vi "application.vi"() -> ()   [LabVIEW 2014, in "application.lvclass"]
uses:
  application.lvclass
  application.lvclass/application.ctl
  <vilib>/Utility/config.llb/NI_LVConfig.lvlib
panel:
  in  "Tab Control":enum32{"Main", "Settings"}(tab)
  in  "Settings":bool
  out "CMD":string caption="命令行"
  in  "file path":path=path "D:/Projects/Personal/Multi-LabVIEW-Selector/Multi-LabVIEW Selector.lvproj" caption="打开文件路径"
  in  "LabVIEW List":string(combo)
  in  "OK":bool
  in  "Cancel":bool
  in  "associate file extension":bool
  in  "System Array":string[](array[string]) caption="File Extension"
  in  "Display Time(ms)":i32 min=0 max=10000 step=100
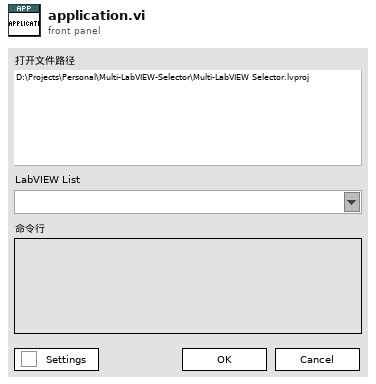
[diagram p1: front panel]
types:
  T1 = enum32{"invalid app kind", "Development System", "Run Time System", "Student Edition", "Embedded LabVIEW", "Evaluation", "Custom"}
  T2 = enum32{"Invalid", "Standard", "Closed", "Hidden", "Minimized", "Maximized"}
  T3 = cluster{"Core":cluster{"Current VI Reference":refnum<vi>, "Close Panel on Exit?":bool}, "RuntimeEngine":bool, "ConfigFilePath":path}
  T4 = cluster{"Current VI Reference":refnum<vi>, "Close Panel on Exit?":bool}
  T5 = typedef "NI_LVConfig.lvlib/Config Data RefNum.ctl" = refnum<k1>
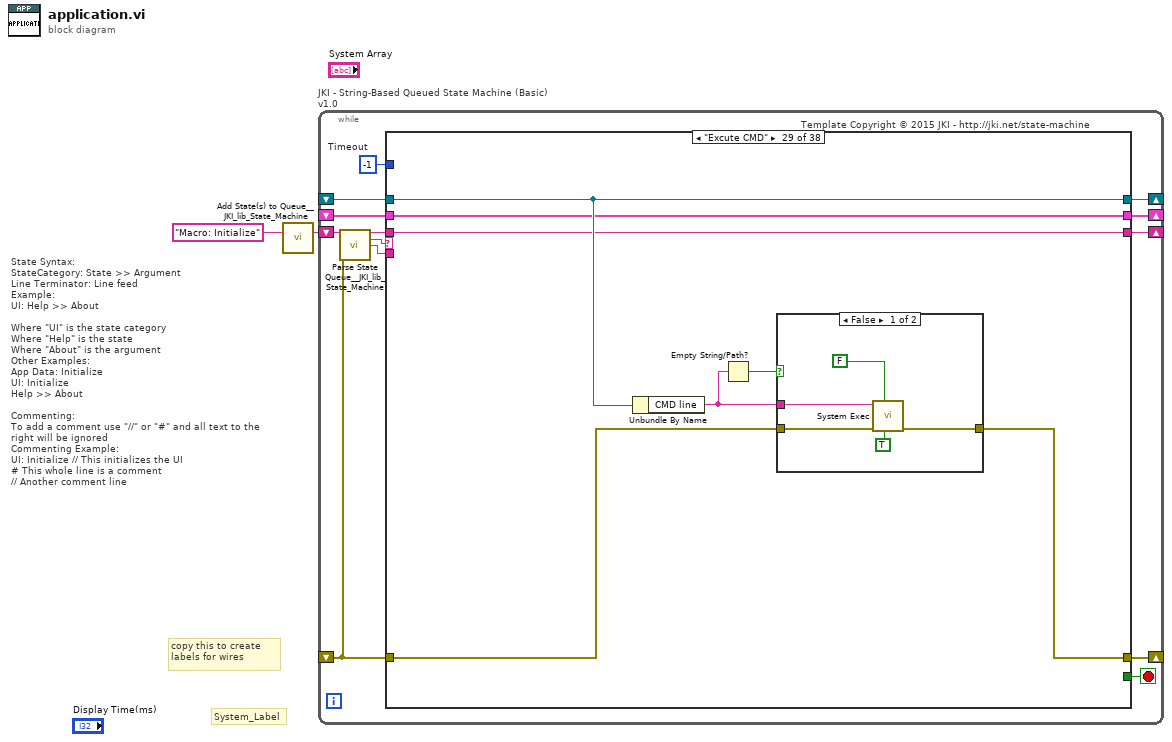
[diagram p0: block diagram]
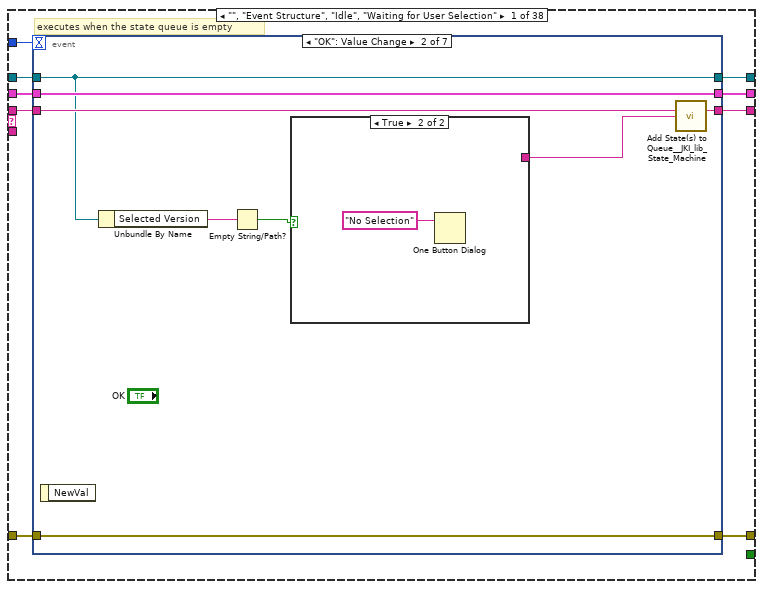
[diagram p2: hidden frame]
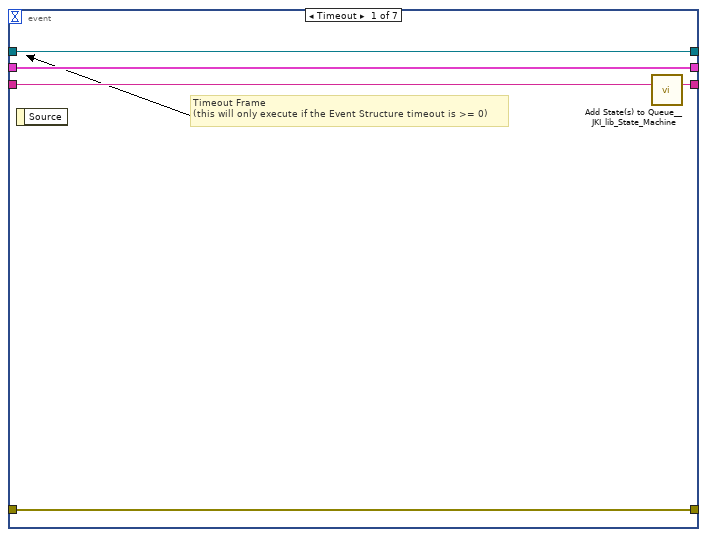
[diagram p3: hidden frame]
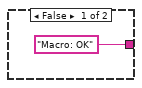
[diagram p4: hidden frame]
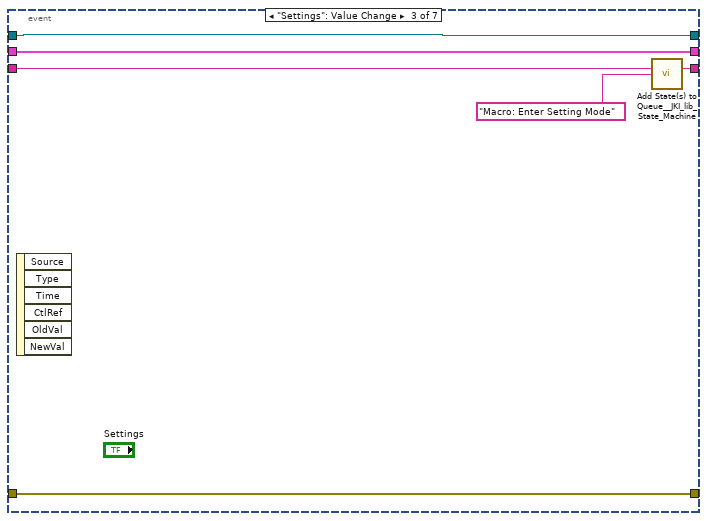
[diagram p5: hidden frame]
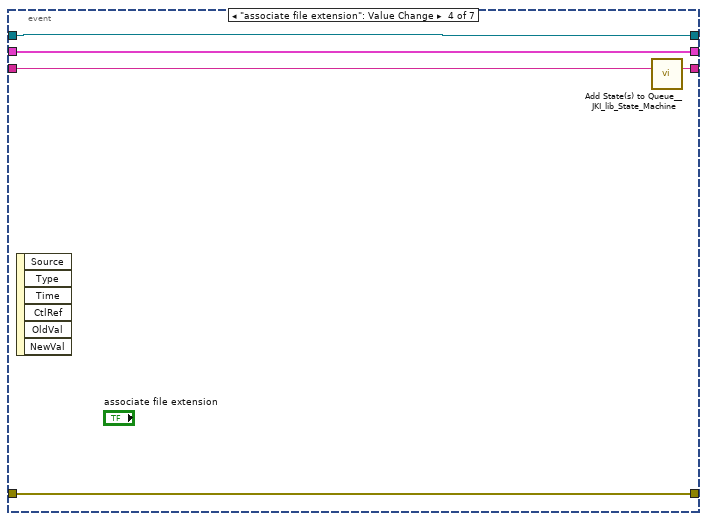
[diagram p6: hidden frame]
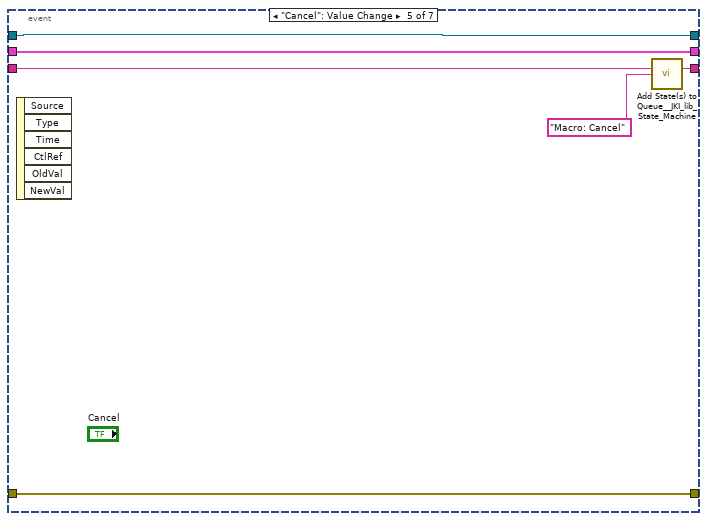
[diagram p7: hidden frame]
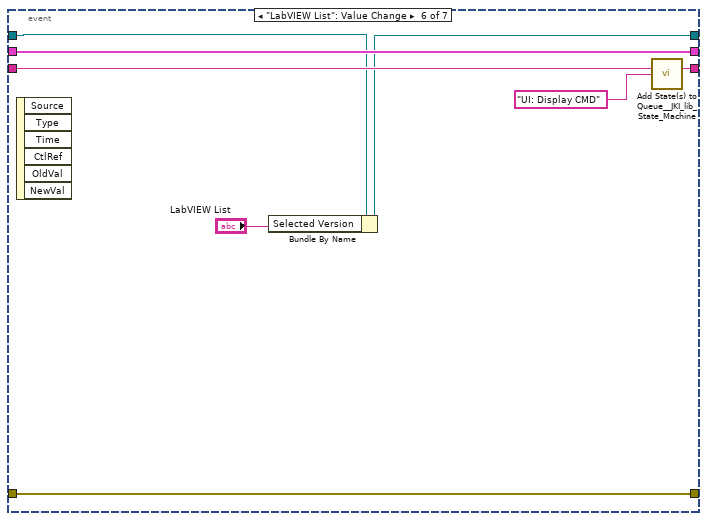
[diagram p8: hidden frame]
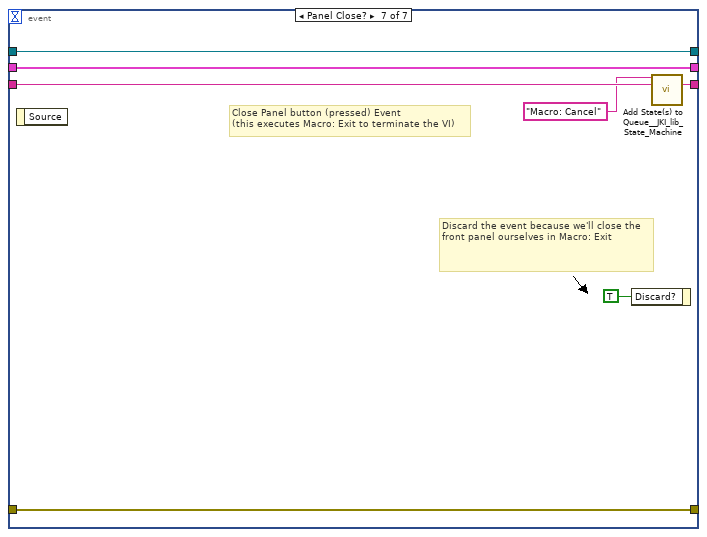
[diagram p9: hidden frame]
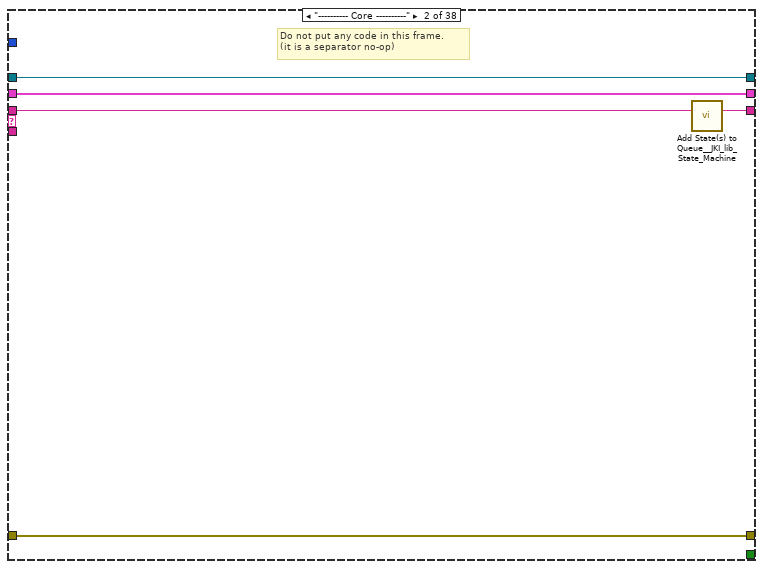
[diagram p10: hidden frame]
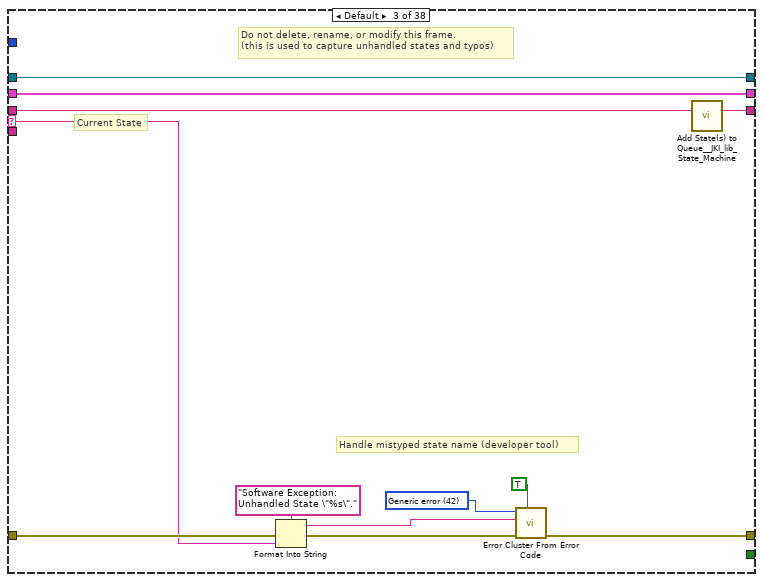
[diagram p11: hidden frame]
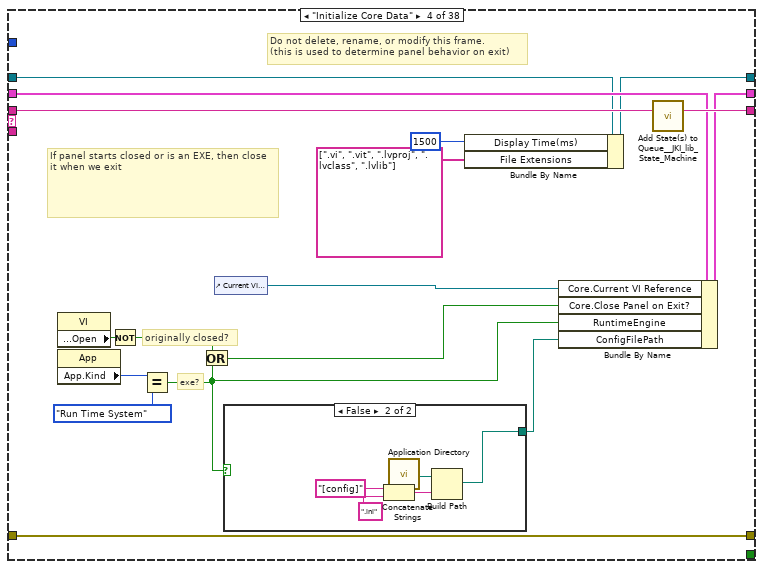
[diagram p12: hidden frame]
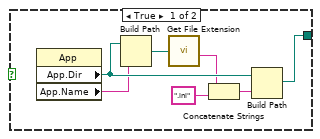
[diagram p13: hidden frame]
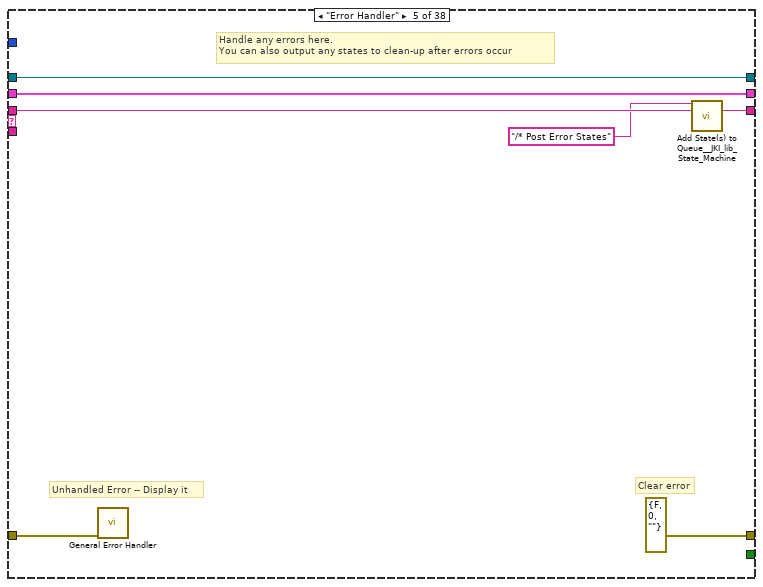
[diagram p14: hidden frame]
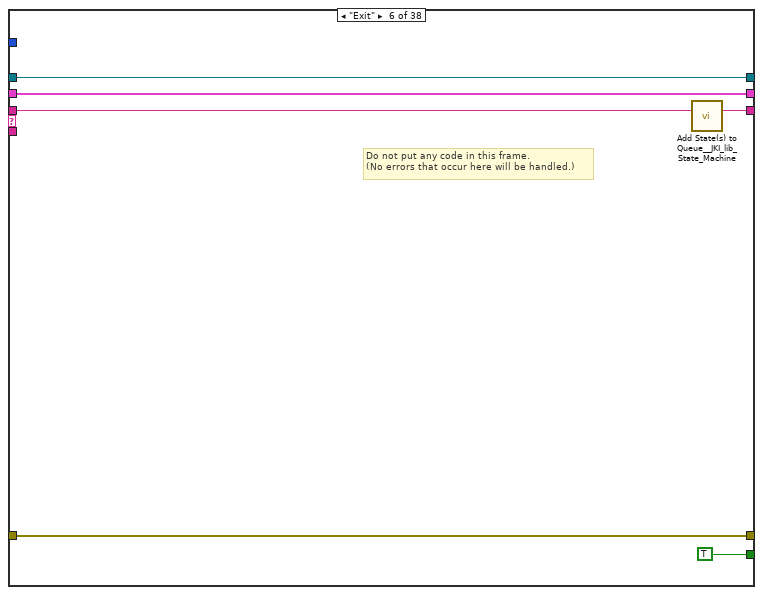
[diagram p15: hidden frame]
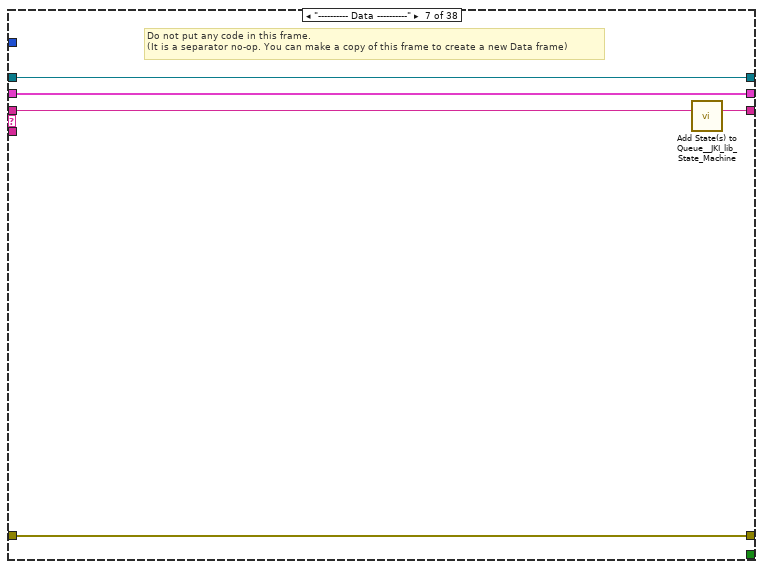
[diagram p16: hidden frame]
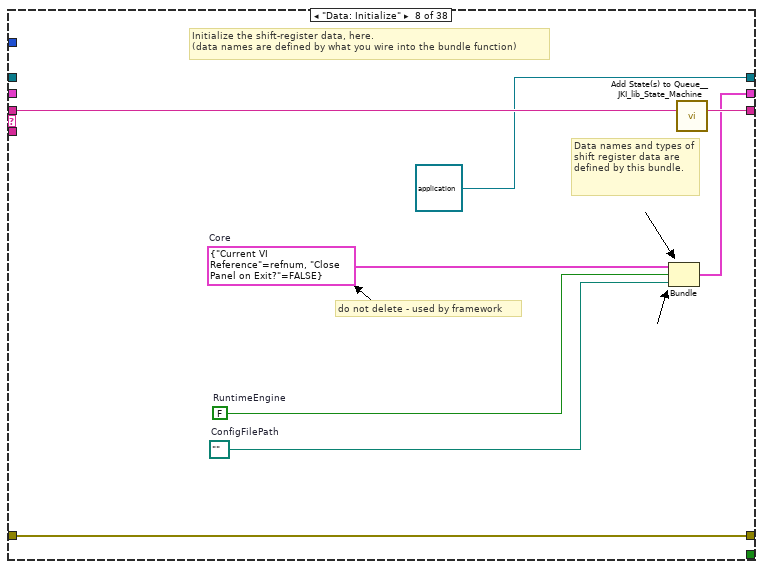
[diagram p17: hidden frame]
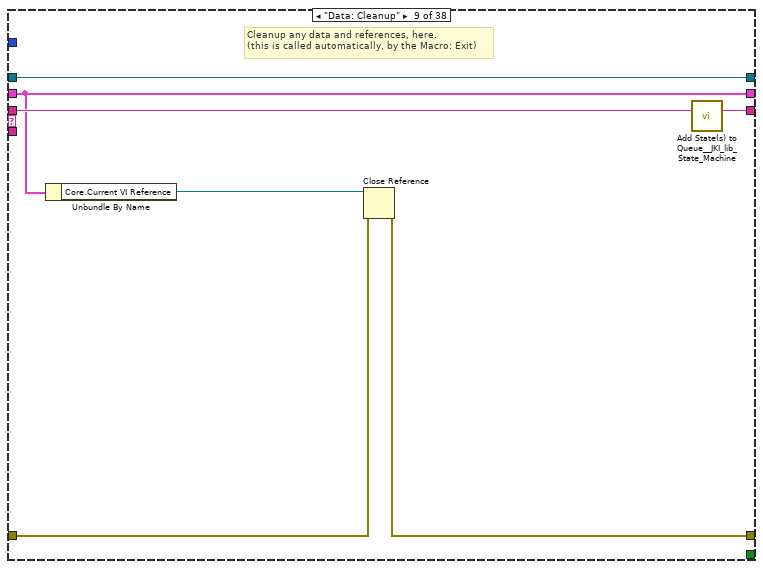
[diagram p18: hidden frame]
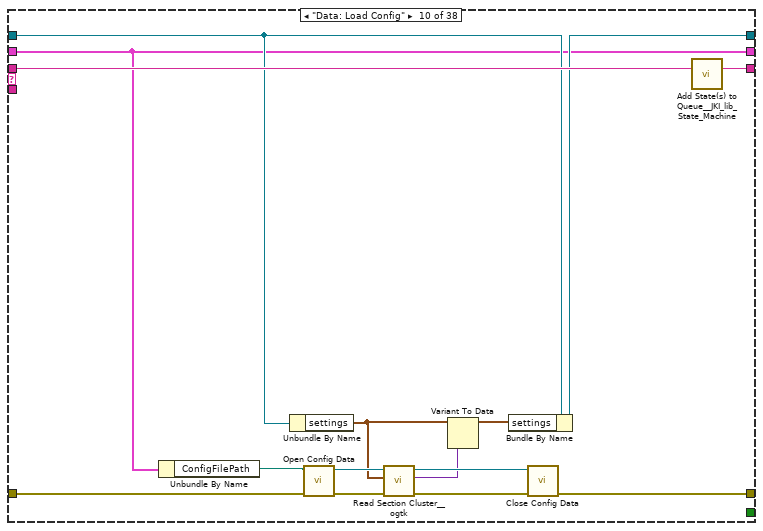
[diagram p19: hidden frame]
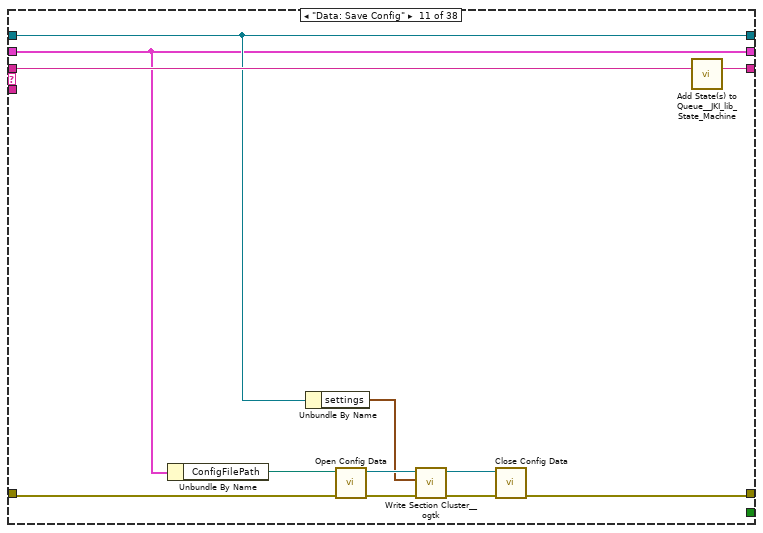
[diagram p20: hidden frame]
diagram:
  # "State Syntax:\nStateCategory: State >> Argument\nLine Terminator: Line feed\nExample:\nUI: Help >> About\n\nWhere \"UI\" is the state category\nWhere \"Help\" is the state\nWhere \"About\" is the argument\nOther Examples:\nApp Data: Initialize\nUI: Initialize\nHelp >> About\n\nCommenting:\nTo add a comment use \"//\" or \"#\" and all text to the right will be ignored\nCommenting Example:\nUI: Initialize // This initializes the UI\n# This whole line is a comment\n// Another comment line"
  # "copy this to create labels for wires"
  # "System_Label"
  n1 = call <vilib>:"Add State(s) to Queue__JKI_lib_State_Machine.vi"("State(s) in (\"\")"="Macro: Initialize") -> ("States Out"=w2:string)  [unwired: 14 in]
  n2 = while "JKI - String-Based Queued State Machine (Basic) v1.0" {
    shift-right: [w8] -> _
    shift-left: _ -> [w7]
    shift-right: [w11] -> _
    shift-left: _ -> [w5]
    shift-right: [w10] -> _
    shift-left: w2 -> [w12]
    shift-right: [w4] -> _
    shift-left: _ -> [w3]
    stop <- w9 stop-if-true
    w6 = -1  # Timeout
    # "Template Copyright © 2015 JKI - http://jki.net/state-machine"
    n3 = call <vilib>:"Parse State Queue__JKI_lib_State_Machine.vi"("State Queue"=w12, "Error In (no error)"=w5) -> ("Remaining States"=w14:string, "Current State"=w15:string, "Arguments"=w13:string)  [unwired: 11 in]
    n4 = case shown="\"Excute CMD\"" w15 {
      selector: w15 -> [_ _ w78 _ _ _ _ _ _ _ _ _ _ _ _ _ _ _ _ _ _ _ _ _ _ _ _ _ _ _ _ _ _ _ _ _ _ _]
      tunnel: w14 -> [w24 w76 w82 w105 w124 w130 w135 w143 w150 w165 w177 w184 w189 w202 w213 w225 w255 w263 w270 w277 w284 w290 w296 w302 w313 w319 w325 w330 w335 w349 w363 w372 w389 w406 w423 w435 w445 w463]
      tunnel: w13 -> [_ _ _ _ _ _ _ _ _ _ _ _ _ _ w208 w219 _ _ _ w272 _ _ _ _ _ _ _ _ _ _ _ _ _ _ _ _ _ _]
      tunnel: w7 -> [w22 w73 w80 w97 w121 w128 w132 _ w145 w152 w166 w182 w186 w200 w211 w221 w253 w260 w267 w274 w281 w287 w293 w299 w310 w316 w322 w327 w336 w345 w360 w368 w391 w408 w425 w437 w447 w465]
      tunnel: [w21 w74 w84 w102 errorcluster {"status"=FALSE, "code"=0, "source"=""} ("error out") w127 w133 w140 w146 w157 w170 w180 w187 w198 w209 w222 w250 w261 w268 w275 w282 w288 w294 w300 w311 w317 w323 w328 w333 w347 w361 w374 w387 w399 w416 w426 w443 w462] -> w11
      tunnel: w5 -> [w20 w74 w83 w102 w120 w127 w133 w140 w147 w158 w169 w181 w187 w196 w210 w223 w251 w261 w268 w275 w282 w288 w294 w300 w311 w317 w323 w328 w334 w348 w361 w375 w387 w400 w417 w427 w444 w462]
      tunnel: [w23 w75 w81 w104 w123 w129 w134 w142 w149 w164 w176 w183 w188 w201 w212 w224 w254 w262 w269 w276 w283 w289 w295 w301 w312 w318 w324 w329 w335 w349 w362 w373 w390 w407 w424 w436 w446 w464] -> w10
      tunnel: [_ _ _ _ _ TRUE _ _ _ _ _ _ _ _ _ _ _ _ _ _ _ _ _ _ _ _ _ _ _ _ _ _ _ _ _ _ _ _] -> w9
      tunnel: [w19 w73 w80 w103 w121 w128 w132 w141 w145 w152 w166 w182 w186 w200 w211 w221 w253 w260 w267 w274 w281 w287 w293 w299 w310 w316 w322 w327 w336 w345 w360 w368 w391 w408 w425 w437 w447 w465] -> w8
      tunnel: w6 -> [w18 _ _ _ _ _ _ _ _ _ _ _ _ _ _ _ _ _ _ _ _ _ _ _ _ _ _ _ _ _ _ _ _ _ _ _ _ _]
      tunnel: [w16 w72 w77 w93 w118 w125 w131 refnum<class "application.lvclass"> refnum ("application.lvclass") w144 w156 w168 w178 w185 w199 w207 w218 w248 w257 w266 w273 w280 w285 w291 w297 w303 w315 w321 w326 w337 w346 w359 w371 w388 w401 w418 w428 w442 w457] -> w4
      tunnel: w3 -> [w17 w72 w77 w94 w118 w125 w131 _ w144 w163 w168 w179 w185 w199 w207 w218 w249 w257 w266 w273 w280 w285 w291 w297 w303 w315 w321 w326 w337 w346 w359 w376 w388 w402 w419 w428 w442 w458]
      frame "", "Event Structure", "Idle", "Waiting for User Selection" {
        # "executes when the state queue is empty"
        n5 = event shown="[1] \"OK\": Value Change" {
          selector: _ -> [_ _ _ _ _ _ _]
          dyn-events: _ -> [_ _ _ _ _ _ _]
          timeout: w18 -> [_ _ _ _ _ _ _]
          tunnel: w24 -> [w29 w37 w45 w50 w56 w64 w71]
          tunnel: [w28 w36 w44 w49 w55 w63 w70] -> w23
          tunnel: w22 -> [w26 w35 w42 w47 w53 w61 w68]
          tunnel: [w27 w34 w43 w48 w54 w62 w69] -> w21
          tunnel: w20 -> [w27 w34 w43 w48 w54 w62 w69]
          tunnel: [w26 w35 w42 w47 w53 w61 w68] -> w19
          tunnel: w17 -> [w25 w33 w41 w46 w52 w60 w65]
          tunnel: [w25 w33 w41 w46 w52 w58 w65] -> w16
          event Timeout {
            # "Timeout Frame\n(this will only execute if the Event Structure timeout is >= 0)"
            n6 = event-data() -> ()  [unwired: 1 in, 1 out]
            n7 = call <vilib>:"Add State(s) to Queue__JKI_lib_State_Machine.vi"("State(s) in (\"\")"=w29) -> ("States Out"=w28:string)  [unwired: 14 in]
          }
          event "OK": Value Change {
            n8 = event-data() -> ()  [unwired: 1 in, 1 out]
            n9 = Unbundle By Name(w33) -> ("Selected Version"=w32:string)
            n10 = Empty String/Path?(string/path=w32) -> (empty?=w31:bool)
            n11 = case shown="True" w31 {
              tunnel: ["Macro: OK" ("State(s) at Back (\"\")") _] -> w30
              frame False {
              }
              frame True {
                n12 = One Button Dialog(message="No Selection") -> ()  [unwired: 1 in, 1 out]
              }
            }
            n13 = call <vilib>:"Add State(s) to Queue__JKI_lib_State_Machine.vi"("State(s) in (\"\")"=w37, "State(s) at Back (\"\")"=w30) -> ("States Out"=w36:string)  [unwired: 13 in]
          }
          event "Settings": Value Change {
            n14 = event-data() -> ()  [unwired: 1 in, 6 out]
            n15 = call <vilib>:"Add State(s) to Queue__JKI_lib_State_Machine.vi"("State(s) in (\"\")"=w45, "State(s) at Back (\"\")"="Macro: Enter Setting Mode" ("State(s) at Back (\"\")")) -> ("States Out"=w44:string)  [unwired: 13 in]
          }
          event "associate file extension": Value Change {
            n16 = event-data() -> ()  [unwired: 1 in, 6 out]
            n17 = call <vilib>:"Add State(s) to Queue__JKI_lib_State_Machine.vi"("State(s) in (\"\")"=w50) -> ("States Out"=w49:string)  [unwired: 14 in]
          }
          event "Cancel": Value Change {
            n18 = event-data() -> ()  [unwired: 1 in, 6 out]
            n19 = call <vilib>:"Add State(s) to Queue__JKI_lib_State_Machine.vi"("State(s) in (\"\")"=w56, "State(s) at Back (\"\")"="Macro: Cancel" ("State(s) at Back (\"\")")) -> ("States Out"=w55:string)  [unwired: 13 in]
          }
          event "LabVIEW List": Value Change {
            n20 = event-data() -> ()  [unwired: 1 in, 6 out]
            n21 = Bundle By Name(cluster=w60, "Selected Version"="LabVIEW List") -> (w58:refnum<class "application.lvclass">)
            n22 = call <vilib>:"Add State(s) to Queue__JKI_lib_State_Machine.vi"("State(s) in (\"\")"=w64, "State(s) at Back (\"\")"="UI: Display CMD" ("State(s) at Back (\"\")")) -> ("States Out"=w63:string)  [unwired: 13 in]
          }
          event Panel Close? {
            # "Discard the event because we'll close the front panel ourselves in Macro: Exit"
            # "Close Panel button (pressed) Event\n(this executes Macro: Exit to terminate the VI)"
            n23 = event-data() -> ()  [unwired: 1 in, 1 out]
            n24 = event-data("Discard?"=TRUE) -> ()  [unwired: 1 in, 1 out]
            n25 = call <vilib>:"Add State(s) to Queue__JKI_lib_State_Machine.vi"("State(s) in Front (\"\")"="Macro: Cancel", "State(s) in (\"\")"=w71) -> ("States Out"=w70:string)  [unwired: 13 in]
          }
        }
      }
      frame "---------- Core ----------" {
        # "Do not put any code in this frame.\n(it is a separator no-op)"
        n26 = call <vilib>:"Add State(s) to Queue__JKI_lib_State_Machine.vi"("State(s) in (\"\")"=w76) -> ("States Out"=w75:string)  [unwired: 14 in]
      }
      frame Default {
        w87 = 42 items=["No error", "Argument error", "Memory is full", "Out of zone", "End of file", "File already open", "Generic file I/O error", "File not found", "File permission error", "Disk is full", "Duplicate path", "Too many files open", "System feature not enabled", "Resource file not found", "Cannot add resource", "Resource not found", "Image not found", "Image memory error", "Pen does not exist", "Config type invalid", "Config token not found", "Config parse error", "Config memory error", "Bad external code format", "Bad external code offset", "External code not present", "Null window", "Destroy window error", "Null menu", "Print aborted", "Bad print record", "Print driver error", "Windows error during printing", "Memory error during printing", "Print dialog error", "Generic print error", "Invalid device refnum", "Device not found", "Device parameter error", "Device unit error", "Cannot open device", "Device call aborted", "Generic error", "Cancelled by user", "Object ID too low", "Object ID too high", "Object not in heap", "Unknown heap", "Unknown object (invalid DefProc)", "Unknown object (DefProc not in table)", "Message out of range", "Invalid (null) method", "Unknown message", "Manager call not supported", "Bad address", "Network operation in progress", "Network operation timed out", "Connection is busy", "Network attribute not supported", "Network error", "Address in use", "System out of memory", "Connection aborted", "Connection refused", "Not connected", "Already connected", "Connection closed", "Initialization error (interapplication manager)", "Bad occurrence", "Wait on unbound occurrence handler", "Occurrence queue overflow", "Datalog type conflict", "Unused", "Unrecognized type (interapplication manager)", "Memory corrupt", "Failed to make temporary DLL", "Old CIN version", "Drag socket not found", "Failed to load drop-object", "Failed to register OLE object", "Failed to release OLE object", "Format specifier type mismatch", "Unknown format specifier", "Too few format specifiers", "Too many format specifiers", "Scan failed", "Newer CIN version", "Error converting to variant", "Runtime menu error", "Password tampered", "Variant attribute not found", "Incompatible variant data type", "Event data is not available", "Event Store is not present", "Occurrence is not found", "Event Queue is not created", "Event info is not available", "Refnum passed is NULL", "Error retrieving Class GUID", "Error retrieving CoClass GUID", "Error retrieving TypeLib GUID.", "Bad built application magic bytes.", "Specific driver is different from the specific driver associated with the Logical Name.", "There is no session opened to the class driver.", "Max Error", "MAX - Error with config objects", "MAX - Error loading configuration", "MAX - Group not supported"]
        # "Current State"
        # "Do not delete, rename, or modify this frame.\n(this is used to capture unhandled states and typos)"
        # "Handle mistyped state name (developer tool)"
        n27 = Format Into String(format string="Software Exception: Unhandled State \"%s\"." ("message"), error in=w83, w78) -> (resulting string=w86:string, error out=w85:errorcluster)  [unwired: 1 in]
        n28 = call <vilib>:"Error Cluster From Error Code.vi"("show call chain? (False)"=TRUE, "error in (no error)"=w85, "error message (\"\")"=w86, "error code (0)"=w87) -> ("error out"=w84:errorcluster)  [unwired: 5 in]
        n29 = call <vilib>:"Add State(s) to Queue__JKI_lib_State_Machine.vi"("State(s) in (\"\")"=w82) -> ("States Out"=w81:string)  [unwired: 14 in]
      }
      frame "Initialize Core Data" {
        # "Do not delete, rename, or modify this frame.\n(this is used to determine panel behavior on exit)"
        # "originally closed?"
        # "exe?"
        # "If panel starts closed or is an EXE, then close it when we exit"
        n30 = property class="VI"() -> ("Front Panel.Open"=w101:bool)  [unwired: 2 in, 2 out]
        n31 = property class="App"() -> ("App.Kind"=w100:T1)  [unwired: 2 in, 2 out]
        n32 = Not(x=w101) -> (.not. x?=w98:bool)
        n33 = Equal?(x=w100, y=T1."Run Time System" ("Application:Kind")) -> (x = y?=w89:bool)
        n34 = Or(x=w98, y=w89) -> (x .or. y?=w96:bool)
        n35 = control-ref of="Current VI Reference"() -> (w95:refnum<vi>)
        n36 = case shown="False" w89 {
          tunnel: [w110 w114] -> w90
          frame True {
            n37 = property class="App"() -> ("App.Dir"=w109:path, "App.Name"=w108:string)  [unwired: 2 in, 2 out]
            n38 = Build Path(base path=w109, name or relative path=w108) -> (appended path=w107:path)
            n39 = call <vilib>:"Get File Extension.vi"("file"=w107) -> ("filename without extension"=w106:string)  [unwired: 7 in, 3 out]
            n40 = Concatenate Strings(w106, ".ini" ("Application:Name")) -> (w111:string)
            n41 = Build Path(base path=w109, name or relative path=w111) -> (appended path=w110:path)
          }
          frame False {
            n42 = Concatenate Strings("[config]" ("string"), ".ini" ("Application:Name")) -> (w115:string)
            n43 = call <vilib>:"Application Directory.vi"() -> ("Application Directory"=w116:path)
            n44 = Build Path(base path=w116, name or relative path=w115) -> (appended path=w114:path)
          }
        }
        n45 = Bundle By Name(cluster=w94, "Display Time(ms)"=1500 ("settings.Display Time(ms)"), "File Extensions"=string[] [".vi", ".vit", ".lvproj", ".lvclass", ".lvlib"]) -> (w93:refnum<class "application.lvclass">)
        n46 = Bundle By Name(cluster=w97, "Core.Current VI Reference"=w95, "Core.Close Panel on Exit?"=w96, "RuntimeEngine"=w89, "ConfigFilePath"=w90) -> (w103:T3)
        n47 = call <vilib>:"Add State(s) to Queue__JKI_lib_State_Machine.vi"("State(s) in (\"\")"=w105) -> ("States Out"=w104:string)  [unwired: 14 in]
      }
      frame "Error Handler" {
        # "Unhandled Error -- Display it"
        # "Handle any errors here.\nYou can also output any states to clean-up after errors occur"
        # "Clear error"
        n48 = call <vilib>:"General Error Handler.vi"("error in (no error)"=w120) -> ()  [unwired: 10 in, 5 out]
        n49 = call <vilib>:"Add State(s) to Queue__JKI_lib_State_Machine.vi"("State(s) in Front (\"\")"="/* Post Error States", "State(s) in (\"\")"=w124) -> ("States Out"=w123:string)  [unwired: 13 in]
      }
      frame "Exit" {
        # "Do not put any code in this frame.\n(No errors that occur here will be handled.)"
        n50 = call <vilib>:"Add State(s) to Queue__JKI_lib_State_Machine.vi"("State(s) in (\"\")"=w130) -> ("States Out"=w129:string)  [unwired: 14 in]
      }
      frame "---------- Data ----------" {
        # "Do not put any code in this frame.\n(It is a separator no-op. You can make a copy of this frame to create a new Data frame)"
        n51 = call <vilib>:"Add State(s) to Queue__JKI_lib_State_Machine.vi"("State(s) in (\"\")"=w135) -> ("States Out"=w134:string)  [unwired: 14 in]
      }
      frame "Data: Initialize" {
        w137 = T4 {"Current VI Reference"=refnum, "Close Panel on Exit?"=FALSE}  # Core
        w139 = FALSE  # RuntimeEngine
        w138 = path ""  # ConfigFilePath
        # "do not delete - used by framework"
        # "Data names and types of shift register data are defined by this bundle."
        # "Initialize the shift-register data, here.\n(data names are defined by what you wire into the bundle function)"
        n52 = Bundle("Core"=w137, "RuntimeEngine"=w139, "ConfigFilePath"=w138) -> (w141:T3)  [unwired: 1 in]
        n53 = call <vilib>:"Add State(s) to Queue__JKI_lib_State_Machine.vi"("State(s) in (\"\")"=w143) -> ("States Out"=w142:string)  [unwired: 14 in]
      }
      frame "Data: Cleanup" {
        # "Cleanup any data and references, here.\n(this is called automatically, by the Macro: Exit)"
        n54 = Unbundle By Name(w145) -> ("Core.Current VI Reference"=w148:refnum<vi>)
        n55 = Close Reference(reference=w148, error in (no error)=w147) -> (error out=w146:errorcluster)
        n56 = call <vilib>:"Add State(s) to Queue__JKI_lib_State_Machine.vi"("State(s) in (\"\")"=w150) -> ("States Out"=w149:string)  [unwired: 14 in]
      }
      frame "Data: Load Config" {
        n57 = Unbundle By Name(w152) -> ("ConfigFilePath"=w151:path)
        n58 = Unbundle By Name(w163) -> ("settings"=w153:cluster{"Display Time(ms)":i32})
        n59 = call <vilib>:"Open Config Data.vi"("error in (no error)"=w158, "configuration file path"=w151) -> ("error out"=w161:errorcluster, "refnum"=w162:T5)  [unwired: 7 in, 1 out]
        n60 = call <userlib>:"Read Section Cluster__ogtk.vi"("error in (no error)"=w161, "Section Formatted Cluster Type"=w153, "refnum"=w162) -> ("error out"=w159:errorcluster, "Section Formatted Cluster"=w154:variant, "dup refnum"=w160:T5)  [unwired: 4 in, 2 out]
        n61 = Variant To Data(type=w153, Variant=w154) -> (data=w155:cluster{"Display Time(ms)":i32})  [unwired: 1 in, 1 out]
        n62 = Bundle By Name(cluster=w163, "settings"=w155) -> (w156:refnum<class "application.lvclass">)
        n63 = call <vilib>:"Close Config Data.vi"("error in (no error)"=w159, "refnum"=w160) -> ("error out"=w157:errorcluster)  [unwired: 8 in, 1 out]
        n64 = call <vilib>:"Add State(s) to Queue__JKI_lib_State_Machine.vi"("State(s) in (\"\")"=w165) -> ("States Out"=w164:string)  [unwired: 14 in]
      }
      frame "Data: Save Config" {
        n65 = Unbundle By Name(w166) -> ("ConfigFilePath"=w167:path)
        n66 = Unbundle By Name(w168) -> ("settings"=w171:cluster{"Display Time(ms)":i32})
        n67 = call <vilib>:"Open Config Data.vi"("error in (no error)"=w169, "configuration file path"=w167) -> ("error out"=w174:errorcluster, "refnum"=w175:T5)  [unwired: 7 in, 1 out]
        n68 = call <userlib>:"Write Section Cluster__ogtk.vi"("error in (no error)"=w174, "Section Formatted Cluster"=w171, "refnum"=w175) -> ("error out"=w172:errorcluster, "dup refnum"=w173:T5)  [unwired: 7 in]
        n69 = call <vilib>:"Close Config Data.vi"("error in (no error)"=w172, "refnum"=w173) -> ("error out"=w170:errorcluster)  [unwired: 8 in, 1 out]
        n70 = call <vilib>:"Add State(s) to Queue__JKI_lib_State_Machine.vi"("State(s) in (\"\")"=w177) -> ("States Out"=w176:string)  [unwired: 14 in]
      }
      frame "Data: Get Installed LabVIEW Version" {
        n71 = call "GetLabVIEWInfos.vi"("error in (no error)"=w181, "application.lvclass"=w179) -> ("error out"=w180:errorcluster, "application.lvclass (dup)"=w178:refnum<class "application.lvclass">)  [unwired: 8 in]
        n72 = call <vilib>:"Add State(s) to Queue__JKI_lib_State_Machine.vi"("State(s) in (\"\")"=w184) -> ("States Out"=w183:string)  [unwired: 14 in]
      }
      frame "---------- UI ----------" {
        # "Do not put any code in this frame.\n(It is a separator no-op. You can make a copy of this frame to create a new UI frame)"
        n73 = call <vilib>:"Add State(s) to Queue__JKI_lib_State_Machine.vi"("State(s) in (\"\")"=w189) -> ("States Out"=w188:string)  [unwired: 14 in]
      }
      frame "UI: Initialize" {
        # "Initialize the User Interface, here.\n(this is called automatically, by the Macro: Init)"
        n74 = disable-structure shown="Default" {
          disable-tunnel: [FALSE ("Tabs Visible?") FALSE ("Tabs Visible?")] -> w195
          disable-tunnel: [w203 w205] -> w194
          disable-tunnel: [w203 w205] -> w193
          frame condition #0 {
            w203 = u32 16777216
          }
          frame condition #1 (active) {
            w205 = u32 16777216
          }
        }
        n75 = property on="Tab Control" class="TabCtl (strict)"(error in=w196, "Tabs Visible?"=w195, "BG Color"=w194, "FG Color"=w193) -> (error out=w191:errorcluster)  [unwired: 1 in, 1 out]
        n76 = property class="VI"(error in=w191, "Front Panel.Title"="Multi-LabVIEW Selector" ("Front Panel Window:Title")) -> (error out=w190:errorcluster)  [unwired: 1 in, 1 out]
        n77 = call <userlib>:"Fit VI window to Content__ogtk.vi"("error in (no error)"=w190, "border spacing (2 px)"=0) -> ("error out"=w198:errorcluster)  [unwired: 4 in, 1 out]
        n78 = call <vilib>:"Add State(s) to Queue__JKI_lib_State_Machine.vi"("State(s) in (\"\")"=w202) -> ("States Out"=w201:string)  [unwired: 14 in]
      }
      frame "UI: Cursor Set" {
        # "Argument"
        # "Set and Unset Cursor Busy.\n(Usage: \"UI: Cursor Set >> Busy|Idle\")"
        n79 = case shown="\"Idle\", Default" w208 {
          tunnel: w210 -> [w215 w217]
          tunnel: [w214 w216] -> w209
          frame "Idle", Default {
            n80 = call <vilib>:"Unset Busy.vi"("error in (no error)"=w215) -> ("error out"=w214:errorcluster)  [unwired: 10 in]
          }
          frame "Busy" {
            n81 = call <vilib>:"Set Busy.vi"("error in (no error)"=w217) -> ("error out"=w216:errorcluster)  [unwired: 9 in, 1 out]
          }
        }
        n82 = call <vilib>:"Add State(s) to Queue__JKI_lib_State_Machine.vi"("State(s) in (\"\")"=w213) -> ("States Out"=w212:string)  [unwired: 14 in]
      }
      frame "UI: Front Panel State" {
        # "Argument"
        # "Set Front Panel Open or Closed\n(Usage: \"UI: Front Panel State >> Open|Close\")"
        n83 = Unbundle By Name(w221) -> ("Core.Current VI Reference"=w220:refnum<vi>)
        n84 = case shown="\"Open\", Default" w219 {
          tunnel: w223 -> [w229 w242]
          tunnel: [w231 w243] -> w222
          tunnel: w220 -> [w230 w240]
          frame "Open", Default {
            n85 = property class="VI"(reference=w230, error in=w229) -> (reference out=w227:refnum<vi>, error out=w228:errorcluster, "Front Panel.Open"=w226:bool)
            n86 = case shown="False" w226 {
              tunnel: [w234 w237] -> w231
              tunnel: w228 -> [w233 w237]
              tunnel: w227 -> [w232 _]
              frame False {
                n87 = invoke class="VI" method="FP.Open"(reference=w232, error in=w233, "Activate"=TRUE, "State"=T2."Standard") -> (error out=w234:errorcluster)  [unwired: 1 in, 4 out]
              }
              frame True {
              }
            }
          }
          frame "Close" {
            n88 = property class="VI"(reference=w240, error in=w242) -> (reference out=w239:refnum<vi>, error out=w241:errorcluster, "Front Panel.Open"=w238:bool)
            n89 = case shown="True" w238 {
              tunnel: [w244 w247] -> w243
              tunnel: w241 -> [w244 w246]
              tunnel: w239 -> [_ w245]
              frame False {
              }
              frame True {
                n90 = invoke class="VI" method="FP.Close"(reference=w245, error in=w246) -> (error out=w247:errorcluster)  [unwired: 1 in, 2 out]
              }
            }
          }
        }
        n91 = call <vilib>:"Add State(s) to Queue__JKI_lib_State_Machine.vi"("State(s) in (\"\")"=w225) -> ("States Out"=w224:string)  [unwired: 14 in]
      }
      frame "UI: Display CMD" {
        n92 = call "GetCMDLine.vi"("error in (no error)"=w251, "application in"=w249) -> ("error out"=w250:errorcluster, "application out"=w248:refnum<class "application.lvclass">)  [unwired: 8 in]
        n93 = Unbundle By Name(w248) -> ("CMD line"=→"CMD":string)
        n94 = call <vilib>:"Add State(s) to Queue__JKI_lib_State_Machine.vi"("State(s) in (\"\")"=w255) -> ("States Out"=w254:string)  [unwired: 14 in]
      }
      frame "UI: Display LabVIEW Information" {
        n95 = Unbundle By Name(w257) -> ("Version List"=w259:string[], "Selected Version"=w258:string)
        n96 = control-ref of="LabVIEW List"() -> (w256:refnum<vi>)
        n97 = property on="Property Node" class="CmbBox"(reference=w256, "Strings[]"=w259, "Value"=w258) -> ()  [unwired: 1 in, 2 out]
        n98 = call <vilib>:"Add State(s) to Queue__JKI_lib_State_Machine.vi"("State(s) in (\"\")"=w263) -> ("States Out"=w262:string)  [unwired: 14 in]
      }
      frame "UI: Display Settings" {
        n99 = Unbundle By Name(w266) -> ("Display Time(ms)"=w265:i32, "File Extensions"=w264:string[])
        n100 = local write "Display Time(ms)"(w265) -> ()
        n101 = local write "System Array"(w264) -> ()
        n102 = call <vilib>:"Add State(s) to Queue__JKI_lib_State_Machine.vi"("State(s) in (\"\")"=w270) -> ("States Out"=w269:string)  [unwired: 14 in]
      }
      frame "UI: Switch Page" {
        n103 = case shown="\"Settings\"" w272 {
          tunnel: [enum32{"Main", "Settings"}."Settings" ("Tab Control") enum32{"Main", "Settings"}."Main" ("Tab Control")] -> w271
          frame "Settings" {
          }
          frame Default {
          }
        }
        n104 = local write "Tab Control"(w271) -> ()
        n105 = call <vilib>:"Add State(s) to Queue__JKI_lib_State_Machine.vi"("State(s) in (\"\")"=w277) -> ("States Out"=w276:string)  [unwired: 14 in]
      }
      frame "---------- Macro ----------" {
        # "Do not put any code in this frame.\n(It is a separator no-op. You can make a copy of this frame to create a new Macro frame)"
        n106 = call <vilib>:"Add State(s) to Queue__JKI_lib_State_Machine.vi"("State(s) in (\"\")"=w284) -> ("States Out"=w283:string)  [unwired: 14 in]
      }
      frame "Macro: Initialize" {
        # "Initialization Macro\n(This is called once, when the VI starts)"
        n107 = call <vilib>:"Add State(s) to Queue__JKI_lib_State_Machine.vi"("State(s) in Front (\"\")"="Data: Initialize\nInitialize Core Data\nData: Load Config\nData: Get Installed LabVIEW Version\nUI: Initialize\nUI: Front Panel State >> Open\nGet Opened File Name\nUI: Display LabVIEW Information\nUI: Display Settings\nUI: Display CMD", "State(s) in (\"\")"=w290) -> ("States Out"=w289:string)  [unwired: 13 in]
      }
      frame "Macro: OK" {
        # "Initialization Macro\n(This is called once, when the VI starts)"
        n108 = call <vilib>:"Add State(s) to Queue__JKI_lib_State_Machine.vi"("State(s) in Front (\"\")"="Update Symbol\nExcute CMD\nMacro: Exit", "State(s) in (\"\")"=w296) -> ("States Out"=w295:string)  [unwired: 13 in]
      }
      frame "Macro: Cancel" {
        # "Initialization Macro\n(This is called once, when the VI starts)"
        n109 = call <vilib>:"Add State(s) to Queue__JKI_lib_State_Machine.vi"("State(s) in Front (\"\")"="Macro: Exit", "State(s) in (\"\")"=w302) -> ("States Out"=w301:string)  [unwired: 13 in]
      }
      frame "Macro: Exit" {
        # "Exit Macro\n(This is called once, when the VI exits)"
        n110 = Unbundle By Name(w310) -> ("Core.Close Panel on Exit?"=w309:bool)
        n111 = Select(t="UI: Front Panel State >> Close", s=w309, f="") -> (s? t:f=w306:string)
        n112 = call <vilib>:"Add State(s) to Queue__JKI_lib_State_Machine.vi"("State(s) in (\"\")"=w306, "State(s) at Back (\"\")"="Data: Save Config\nData: Cleanup\nExit") -> ("States Out"=w304:string)  [unwired: 13 in]
        n113 = call <vilib>:"Add State(s) to Queue__JKI_lib_State_Machine.vi"("State(s) in Front (\"\")"=w304, "State(s) in (\"\")"=w313) -> ("States Out"=w312:string)  [unwired: 13 in]
      }
      frame "Macro: Enter Setting Mode" {
        n114 = call <vilib>:"Add State(s) to Queue__JKI_lib_State_Machine.vi"("State(s) in Front (\"\")"="UI: Switch Page >> Settings" ("State(s) in Front (\"\")"), "State(s) in (\"\")"=w319) -> ("States Out"=w318:string)  [unwired: 13 in]
      }
      frame "Macro: Enter Normal Mode" {
        n115 = call <vilib>:"Add State(s) to Queue__JKI_lib_State_Machine.vi"("State(s) in Front (\"\")"="UI: Switch Page >> Normal\nFind Symbol\nCheck If The Symbol Version Exist" ("State(s) in Front (\"\")"), "State(s) in (\"\")"=w325) -> ("States Out"=w324:string)  [unwired: 13 in]
      }
      frame "---------- State Machine ----------" {
        n116 = call <vilib>:"Add State(s) to Queue__JKI_lib_State_Machine.vi"("State(s) in (\"\")"=w330) -> ("States Out"=w329:string)  [unwired: 14 in]
      }
      frame "Excute CMD" {
        n117 = Unbundle By Name(w337) -> ("CMD line"=w331:string)
        n118 = Empty String/Path?(string/path=w331) -> (empty?=w332:bool)
        n119 = case shown="False" w332 {
          tunnel: w331 -> [w340 _]
          tunnel: w334 -> [w339 w343]
          tunnel: [w338 w343] -> w333
          frame False {
            n120 = call <vilib>:"System Exec.vi"("run minimized? (F)"=TRUE, "wait until completion? (T)"=FALSE, "error in (no error)"=w339, "command line"=w340) -> ("error out"=w338:errorcluster)  [unwired: 4 in, 3 out]
          }
          frame True {
          }
        }
      }
      frame "Associate with File Extension" {
        n121 = Unbundle By Name(w345) -> ("RuntimeEngine"=w344:bool)
        n122 = case shown="True" w344 {
          tunnel: w348 -> [w350 w354]
          tunnel: [w350 w353] -> w347
          tunnel: w346 -> [_ w352]
          frame False {
          }
          frame True {
            n123 = Unbundle By Name(w352) -> ("File Extensions"=w351:string[])
            n124 = for {
              tunnel: w354 -> [w358]
              tunnel: [w357] -> w353
              tunnel: w351 -> [w356] mode=indexing
              n125 = call "Associate a File Extension.vi"("error in (no error)"=w358, "string"=w356, "exe path"=path "") -> ("error out"=w357:errorcluster)  [unwired: 8 in]
            }
          }
        }
      }
      frame "---------- Actions ----------" {
        n126 = call <vilib>:"Add State(s) to Queue__JKI_lib_State_Machine.vi"("State(s) in (\"\")"=w363) -> ("States Out"=w362:string)  [unwired: 14 in]
      }
      frame "Get Opened File Name" {
        n127 = Unbundle By Name(w368) -> ("RuntimeEngine"=w369:bool)
        n128 = case shown="False" w369 {
          tunnel: w375 -> [w377 w385]
          tunnel: [w377 w384] -> w374
          tunnel: ["file path" w383] -> w370
          tunnel: [FALSE w382] -> w367
          frame False {
          }
          frame True {
            n129 = property class="App"(error in=w385) -> (error out=w384:errorcluster, "App.Args"=w381:string[])  [unwired: 1 in, 1 out]
            n130 = Index Array(array=w381) -> (element #2=w380:string)  [unwired: 2 in, 1 out]
            n131 = String To Path(string=w380) -> (path=w383:path)
            n132 = Empty String/Path?(string/path=w383) -> (empty?=w382:bool)
          }
        }
        n133 = Bundle By Name(cluster=w376, "File Path"=w370) -> (w371:refnum<class "application.lvclass">)
        n134 = Select(t="Macro: Enter Setting Mode", s=w367, f="Macro: Enter Normal Mode") -> (s? t:f=w364:string)
        n135 = call <vilib>:"Add State(s) to Queue__JKI_lib_State_Machine.vi"("State(s) in Front (\"\")"=w364, "State(s) in (\"\")"=w372) -> ("States Out"=w373:string)  [unwired: 13 in]
      }
      frame "Find Symbol" {
        n136 = call <vilib>:"Add State(s) to Queue__JKI_lib_State_Machine.vi"("State(s) in Front (\"\")"="Find New Symbol" ("State(s) at Back (\"\")"), "State(s) in (\"\")"=w389) -> ("States Out"=w390:string)  [unwired: 13 in]
      }
      frame "Find New Symbol" {
        n137 = Unbundle By Name(w402) -> ("File Path"=w405:path)
        n138 = Strip Path(path=w405) -> (stripped path=w393:path)  [unwired: 1 out]
        n139 = call "FindSymbol.vi"("error in (no error)"=w400, "pattern"="DEV ENVIRONMENT *" ("prefix"), "path"=w393) -> ("error out"=w399:errorcluster, "Version"=w404:string, "Exits?"=w392:bool, "Symbol path"=w394:path)  [unwired: 4 in, 1 out]
        n140 = Select(t=w394, s=w392, f=w393) -> (s? t:f=w395:path)
        n141 = Bundle By Name(cluster=w402, "Symbol Path"=w395, "Symbol Version"=w404, "Symbol Found?"=w392) -> (w401:refnum<class "application.lvclass">)
        n142 = Select(t="", s=w392, f="Find Old Symbol" ("State(s) at Back (\"\")")) -> (s? t:f=w396:string)
        n143 = call <vilib>:"Add State(s) to Queue__JKI_lib_State_Machine.vi"("State(s) in Front (\"\")"=w396, "State(s) in (\"\")"=w406) -> ("States Out"=w407:string)  [unwired: 13 in]
      }
      frame "Find Old Symbol" {
        # "If old symbol is found, replace with new symbol."
        n144 = Unbundle By Name(w419) -> ("File Path"=w422:path)
        n145 = Strip Path(path=w422) -> (stripped path=w412:path)  [unwired: 1 out]
        n146 = call "FindSymbol.vi"("error in (no error)"=w417, "pattern"="开发环境 *" ("prefix"), "path"=w412) -> ("error out"=w416:errorcluster, "Version"=w421:string, "Exits?"=w409:bool, "Symbol path"=w410:path)  [unwired: 4 in, 1 out]
        n147 = Select(t=w410, s=w409, f=w412) -> (s? t:f=w411:path)
        n148 = Bundle By Name(cluster=w419, "Symbol Path"=w411, "Symbol Version"=w421, "Symbol Found?"=w409) -> (w418:refnum<class "application.lvclass">)
        n149 = Select(t="Replace with New Symbol", s=w409, f="" ("State(s) at Back (\"\")")) -> (s? t:f=w413:string)
        n150 = call <vilib>:"Add State(s) to Queue__JKI_lib_State_Machine.vi"("State(s) in Front (\"\")"=w413, "State(s) in (\"\")"=w423) -> ("States Out"=w424:string)  [unwired: 13 in]
      }
      frame "Replace with New Symbol" {
        n151 = Unbundle By Name(w428) -> ("Symbol Version"=w430:string, "Symbol Path"=w434:path)
        n152 = call "DeleteSymbolsInDir.vi"("error in (no error)"=w427, "pattern"="开发环境 *", "dup path"=w434) -> ("error in (no error) (dup)"=w432:errorcluster, "dup path (dup)"=w431:path)  [unwired: 7 in]
        n153 = call "CreateSymbolInDir.vi"("error in"=w432, "prefix"="DEV ENVIRONMENT", "Name"=w430, "Path"=w431) -> ("error out"=w426:errorcluster)  [unwired: 6 in, 1 out]
        n154 = call <vilib>:"Add State(s) to Queue__JKI_lib_State_Machine.vi"("State(s) in (\"\")"=w435) -> ("States Out"=w436:string)  [unwired: 14 in]
      }
      frame "Update Symbol" {
        n155 = Unbundle By Name(w442) -> ("Symbol Version"=w440:string, "Selected Version"=w439:string, "Symbol Path"=w441:path)
        n156 = Not Equal?(x=w440, y=w439) -> (x != y?=w438:bool)
        n157 = case shown="True" w438 {
          tunnel: w444 -> [w448 w449]
          tunnel: [w448 w456] -> w443
          tunnel: w441 -> [_ w453]
          tunnel: w439 -> [_ w455]
          frame False {
          }
          frame True {
            n158 = call "DeleteSymbolsInDir.vi"("error in (no error)"=w449, "pattern"="DEV ENVIRONMENT*" ("prefix"), "dup path"=w453) -> ("error in (no error) (dup)"=w450:errorcluster, "dup path (dup)"=w452:path)  [unwired: 7 in]
            n159 = call "CreateSymbolInDir.vi"("error in"=w450, "prefix"="DEV ENVIRONMENT", "Name"=w455, "Path"=w452) -> ("error out"=w456:errorcluster)  [unwired: 6 in, 1 out]
          }
        }
        n160 = call <vilib>:"Add State(s) to Queue__JKI_lib_State_Machine.vi"("State(s) in (\"\")"=w445) -> ("States Out"=w446:string)  [unwired: 14 in]
      }
      frame "Check If The Symbol Version Exist" {
        n161 = Unbundle By Name(w458) -> ("Symbol Found?"=w461:bool, "Version List"=w459:string[], "Symbol Version"=w460:string)
        n162 = case shown="True" w461 {
          tunnel: w459 -> [_ w471]
          tunnel: w460 -> [_ w467]
          tunnel: w458 -> [w466 w469]
          tunnel: [w466 w468] -> w457
          frame False {
          }
          frame True {
            n163 = Search 1D Array(1D array=w471, element=w467) -> (index of element=w472:i32)  [unwired: 1 in]
            n164 = Less Than 0?(x=w472) -> (x < 0?=w470:bool)
            n165 = case shown="True" w470 {
              frame False {
              }
              frame True {
                n166 = One Button Dialog(message="The Symbol Version does not exist on this computer.") -> ()  [unwired: 1 in, 1 out]
              }
            }
            n167 = Bundle By Name(cluster=w469, "Selected Version"=w467) -> (w468:refnum<class "application.lvclass">)
          }
        }
        n168 = call <vilib>:"Add State(s) to Queue__JKI_lib_State_Machine.vi"("State(s) in (\"\")"=w463) -> ("States Out"=w464:string)  [unwired: 14 in]
      }
    }
  }
